vi "ctrlPath.vi"(2 "psi_r":dbl, 3 "psi":dbl) -> (18 "e_psi":dbl)   [LabVIEW 2014]
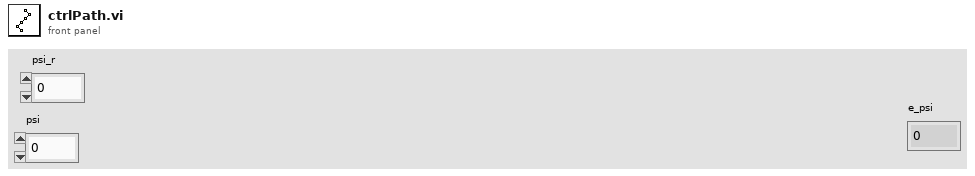
[diagram p1: front panel]
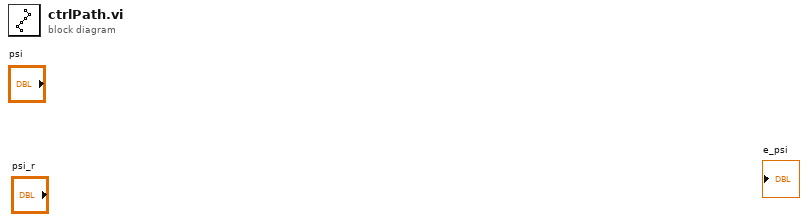
[diagram p0: block diagram]
diagram:
